vi "14_2b.vi"() -> ()   [LabVIEW 2018]
panel:
  out "sum":u64
  out "array":string[](array[string])
  in  "Input":string
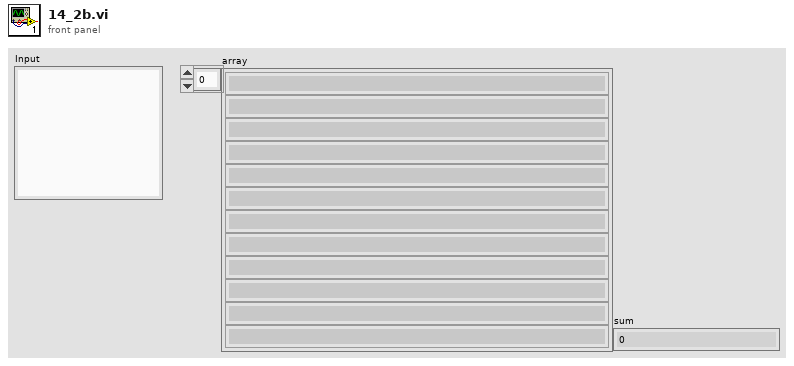
[diagram p1: front panel]
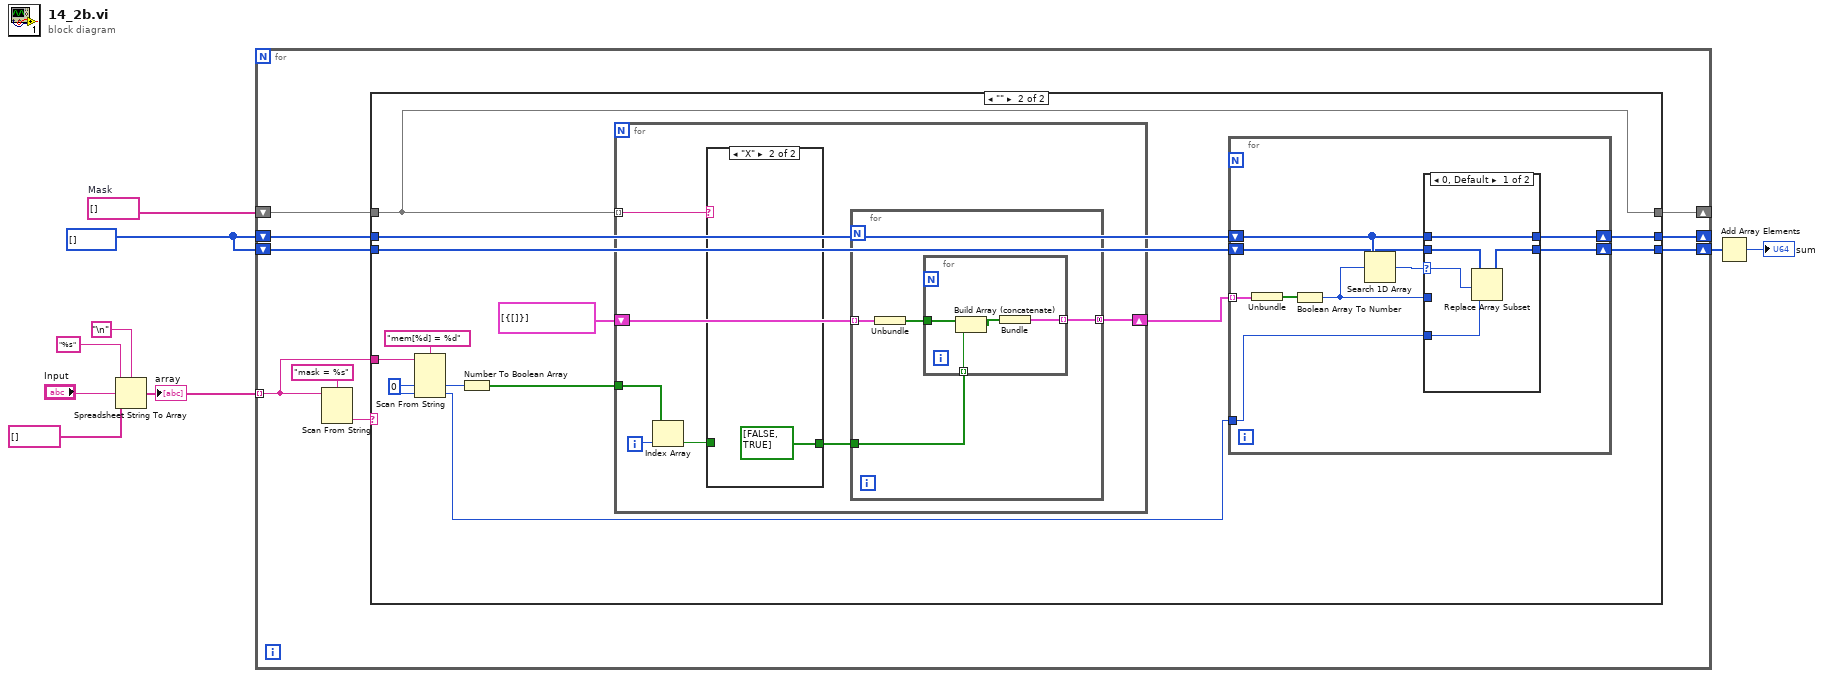
[diagram p0: block diagram]
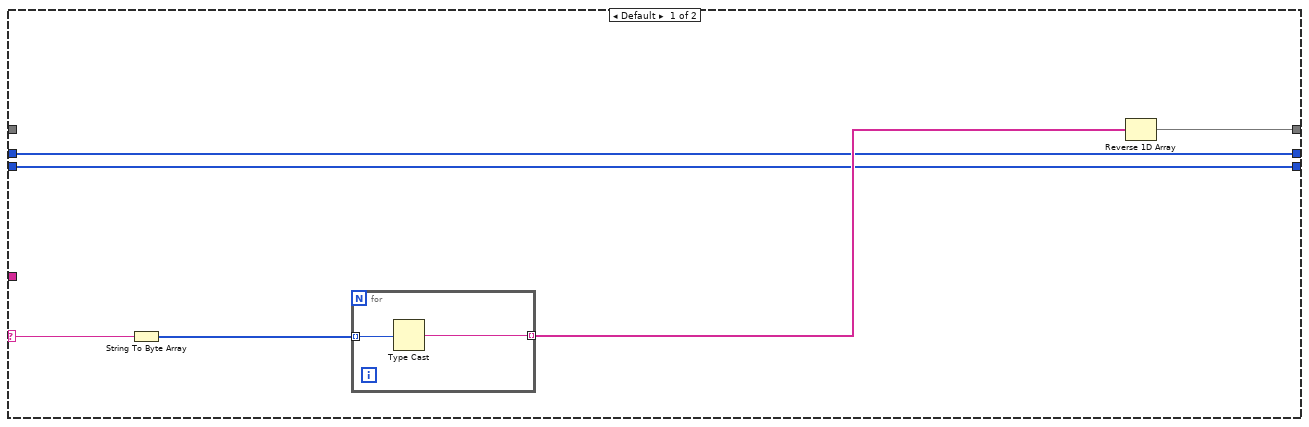
[diagram p2: hidden frame]
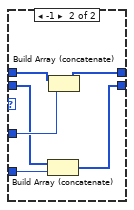
[diagram p3: hidden frame]
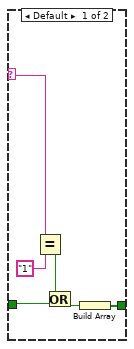
[diagram p4: hidden frame]
diagram:
  w1 = u64[] []
  w4 = string[] []  # Mask
  n1 = Spreadsheet String To Array(delimiter (Tab)="\n", format string="%s", spreadsheet string="Input", array type (2D Dbl)=string[] []) -> (array=w5:string[])
  "array" <- w5
  n2 = for {
    tunnel: w5 -> [w12] mode=indexing
    shift-right: [w15] -> _
    shift-left: w4 -> [w16]
    shift-right: [w13] -> _
    shift-left: w1 -> [w14]
    shift-right: [w10] -> w2
    shift-left: w1 -> [w11]
    n3 = Scan From String(format string="mask = %s", input string=w12) -> (output 1=w17:string)  [unwired: 3 in, 3 out]
    n4 = case shown="\"\"" w17 {
      selector: w17 -> [w24 _]
      tunnel: w16 -> [_ w36]
      tunnel: [w20 w36] -> w15
      tunnel: w14 -> [w21 w35]
      tunnel: [w21 w37] -> w13
      tunnel: w12 -> [_ w39]
      tunnel: w11 -> [w19 w28]
      tunnel: [w19 w27] -> w10
      frame Default {
        n5 = String To Byte Array(string=w24) -> (unsigned byte array=w23:u8[])
        n6 = for {
          tunnel: w23 -> [w26] mode=indexing
          tunnel: [w25] -> w22 mode=indexing
          n7 = Type Cast(x=w26) -> (*(type *) &x=w25:string)  [unwired: 1 in]
        }
        n8 = Reverse 1D Array(array=w22) -> (reversed array=w20:string[])
      }
      frame "" {
        w33 = u64 0
        n9 = Scan From String(format string="mem[%d] = %d", input string=w39, default 1=w33, default 2=w33) -> (output 1=w32:u64, output 2=w34:u64)  [unwired: 2 in, 3 out]
        n10 = Number To Boolean Array(number=w32) -> (Boolean array=w31:bool[])
        n11 = for {
          tunnel: w36 -> [w66] mode=indexing
          shift-right: [w60] -> w29
          shift-left: cluster{bool[]}[] [{[]}] -> [w62]
          tunnel: w31 -> [w63]
          i -> [w64]
          n12 = Index Array(array=w63, index=w64) -> (element=w65:bool)
          n13 = case shown="\"X\"" w66 {
            selector: w66 -> [w80 _]
            tunnel: [w75 bool[] [FALSE, TRUE]] -> w61
            tunnel: w65 -> [w78 _]
            frame Default {
              n14 = Equal?(x=w80, y="1") -> (x = y?=w77:bool)
              n15 = Or(x=w77, y=w78) -> (x .or. y?=w76:bool)
              n16 = Build Array(w76) -> (w75:bool[])
            }
            frame "X" {
            }
          }
          n17 = for {
            tunnel: w62 -> [w70] mode=indexing
            tunnel: w61 -> [w69]
            tunnel: [w67] -> w60 mode=concatenating
            n18 = Unbundle(w70) -> (w68:bool[])
            n19 = for {
              tunnel: w68 -> [w74]
              tunnel: w69 -> [w73] mode=indexing
              tunnel: [w71] -> w67 mode=indexing
              n20 = Build Array (concatenate)(w74, w73) -> (w72:bool[])
              n21 = Bundle(w72) -> (w71:cluster{bool[]})  [unwired: 1 in]
            }
          }
        }
        n22 = for {
          shift-right: [w42] -> w37
          shift-left: w35 -> [w44]
          tunnel: w34 -> [w48]
          tunnel: w29 -> [w47] mode=indexing
          shift-right: [w40] -> w27
          shift-left: w28 -> [w41]
          n23 = Unbundle(w47) -> (w46:bool[])
          n24 = Boolean Array To Number(Boolean array=w46) -> (number=w43:u64)
          n25 = Search 1D Array(1D array=w44, element=w43) -> (index of element=w45:i32)  [unwired: 1 in]
          n26 = case shown="0, Default" w45 {
            selector: w45 -> [w51 _]
            tunnel: w44 -> [w53 w59]
            tunnel: w43 -> [_ w58]
            tunnel: [w53 w57] -> w42
            tunnel: w48 -> [w50 w56]
            tunnel: w41 -> [w52 w55]
            tunnel: [w49 w54] -> w40
            frame 0, Default {
              n27 = Replace Array Subset(array=w52, new element=w50, index=w51) -> (w49:u64[])
            }
            frame -1 {
              n28 = Build Array (concatenate)(w55, w56) -> (w54:u64[])
              n29 = Build Array (concatenate)(w59, w58) -> (w57:u64[])
            }
          }
        }
      }
    }
  }
  n30 = Add Array Elements(numeric array=w2) -> (sum=→"sum":u64)
